vi "CreateTag25h9.vi"(8 "error in (no error)":errorcluster, 11 "Detector Settings":T1={"Refine Edges (Default: True)"=TRUE, "Threads (Default: 1)"=1, "Decimate (Default: 1)"=1.0, "Blur (Default: 0)"=0.0, "Bits (Default: 2)"=2} {"Threads (Default: 1)" min=1}) -> (0 "error out":errorcluster, 3 "New ApriltagDetector":refnum<class "AprilTagDetector.lvclass">)   [LabVIEW 2020, in "g_ar_toolkit.feature_detection.lvlib" / "AprilTagDetector.lvclass"]
uses:
  AprilTagDetector.lvclass
  Detector Settings.ctl
  AprilTag Families.ctl
  AprilTagDetector.lvclass/AprilTagDetector.ctl
  g_ar_toolkit.common/Module Path.vi
  <vilib>/Utility/error.llb/Error Cluster From Error Code.vi
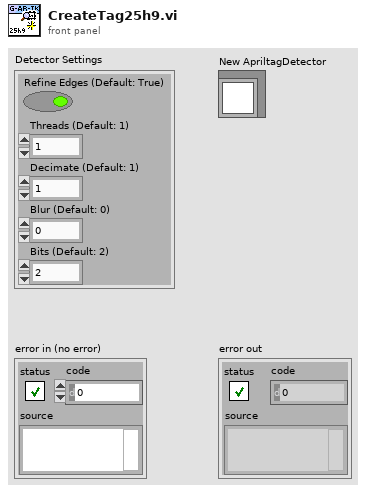
[diagram p1: front panel]
types:
  T1 = typedef "g_ar_toolkit.feature_detection.lvlib/AprilTagDetector.lvclass/Detector Settings.ctl" = cluster{"Refine Edges (Default: True)":bool, "Threads (Default: 1)":u8, "Decimate (Default: 1)":sgl, "Blur (Default: 0)":sgl, "Bits (Default: 2)":u8}
  T2 = typedef "g_ar_toolkit.feature_detection.lvlib/AprilTagDetector.lvclass/AprilTag Families.ctl" = enum8{"tag16h5", "tag25h9", "tag36h11", "tagCircle21h7", "tagCircle49h12", "tagCustom48h12", "tagStandard41h12", "tagStandard52h13"}
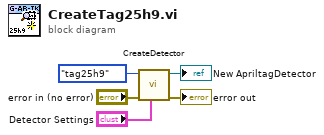
[diagram p0: block diagram]
diagram:
  n1 = call "CreateDetector.vi"("Detector Settings"="Detector Settings", "error in (no error)"="error in (no error)", "Family"=AprilTag_Families."tag25h9") -> ("error out"=→"error out":errorcluster, "New ApriltagDetector"=→"New ApriltagDetector":refnum<class "AprilTagDetector.lvclass">)  [unwired: 7 in]
